vi "temalab 1.vi"() -> ()   [LabVIEW 2021]
uses:
  <vilib>/Math Plots/2D Math Plots/2D Compass/2D Compass XCtrl/2D Compass.xctl
  <vilib>/Math Plots/2D Math Plots/2D Compass/2D Compass Datatype/Public/Plot Helper (Vector).vi
  <vilib>/Instr/_visa.llb/VISA Configure Serial Port (Instr).vi
  <vilib>/Math Plots/2D Math Plots/2D Compass/2D Compass Datatype/2D Compass Datatype.lvclass
panel:
  in  "OK Button":bool
  out "String":string
  out "2D Compass":refnum<class "2D Plot Datatype.lvclass">[](xcontrol)
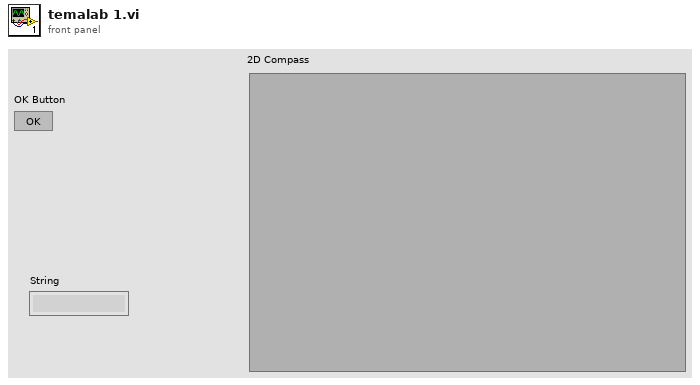
[diagram p1: front panel]
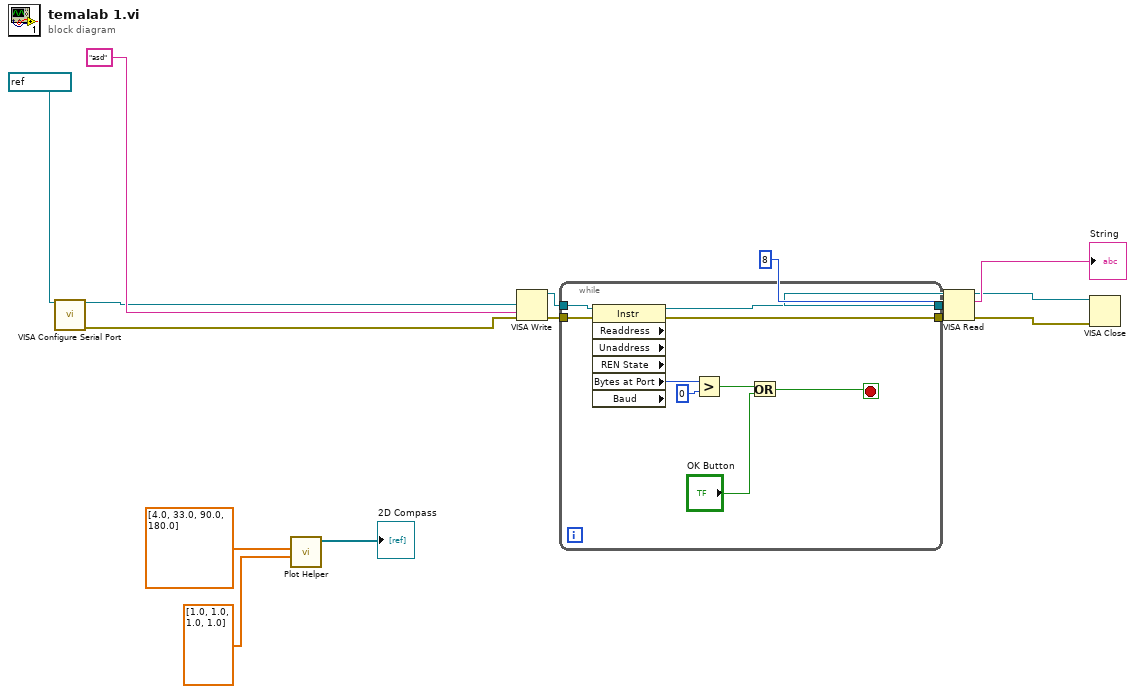
[diagram p0: block diagram]
diagram:
  n1 = call-poly "VISA Configure Serial Port"("VISA resource name"=refnum<visa-resource-name> "COM3") -> ("VISA resource name out"=w6:refnum<visa-resource-name>, "error out"=w5:errorcluster)  [unwired: 13 in]
  n2 = call-poly <vilib>:"Plot Helper.vi"("radius vector"=dbl[] [1.0, 1.0, 1.0, 1.0], "theta vector"=dbl[] [4.0, 33.0, 90.0, 180.0]) -> ("2D Plot Class Obj Array out"=→"2D Compass":refnum<class "2D Plot Datatype.lvclass">[])  [unwired: 2 in, 7 out]
  n3 = VISA Write(VISA resource name=w6, write buffer="asd", error in (no error)=w5) -> (VISA resource name out=w4:refnum<visa-resource-name>, error out=w3:errorcluster)  [unwired: 1 out]
  n4 = while {
    tunnel: w4 -> [w24]
    tunnel: w3 -> [w23]
    tunnel: [w22] -> w2
    tunnel: [w21] -> w1
    stop <- w16 stop-if-true
    n5 = property class="Instr" props=["Readdress", "Unaddress", "REN State", "Bytes at Port", "Baud"](reference=w24, error in=w23) -> (reference out=w22:refnum<visa-resource-name>, error out=w21:errorcluster, "Bytes at Port"=w20:u32)  [unwired: 4 out]
    n6 = Greater?(x=w20, y=0) -> (0:w18:bool)
    n7 = Or(x=w18, y="OK Button") -> (x .or. y?=w16:bool)
  }
  n8 = VISA Read(VISA resource name=w2, byte count=u32 8, error in (no error)=w1) -> (VISA resource name out=w11:refnum<visa-resource-name>, read buffer=→"String":string, error out=w10:errorcluster)  [unwired: 1 out]
  n9 = VISA Close(VISA resource name=w11, error in (no error)=w10) -> ()  [unwired: 1 out]
